vi "RunMeOld.vi"() -> ()   [LabVIEW 2011]
doc: "Use this template to create an application that executes repeatedly until you click the Stop button. This template polls the state of the Stop button and does not use events. Use the Top-Level Application template (not available in the Base package) to create a single-loop application with event handling."
uses:
  Instance           1 33Saved   SingleLoopApplication.vit .vi
  <vilib>/Instr/_visa.llb/VISA Configure Serial Port (Instr).vi
  <vilib>/gmath/NI_Gmath.lvlib
  <vilib>/gmath/NumericalOptimization/Nonlinear Curve Fit LM formula string.vi
panel:
  out "Position":dbl(knob) max=500.0 scale=0.0..360.0
  out "Measurement OK":bool
  out "Residuals":cluster{u32[], dbl[]}(graph)
  out "Instant data":cluster{"velocity":dbl, "position":u32}
  in  "initial parameters":dbl[](array[numeric])=[1.0, 1.0, 1.0]
  out "best fit parameters":dbl[](array[numeric])
  in  "model description":T1={"model"="r+n*sin(x/500*2*3.141593+f)", "Parameters"=["r", "n", "f"], "x"="x"}
  in  "Clear":bool
  in  "index (page)":i32
  out "Previus measurements":cluster{u32[], "best nonlinear fit":dbl[]}[](graph)
  out "Current measurement":cluster{u32[], dbl[]}(graph)
  out "home?":bool=TRUE
  in  "Motor on":bool
  in  "Connect":bool
  in  "VISA resource name":refnum<visa-resource-name>="COM5"
  out "error out":errorcluster
  in  "stop":bool
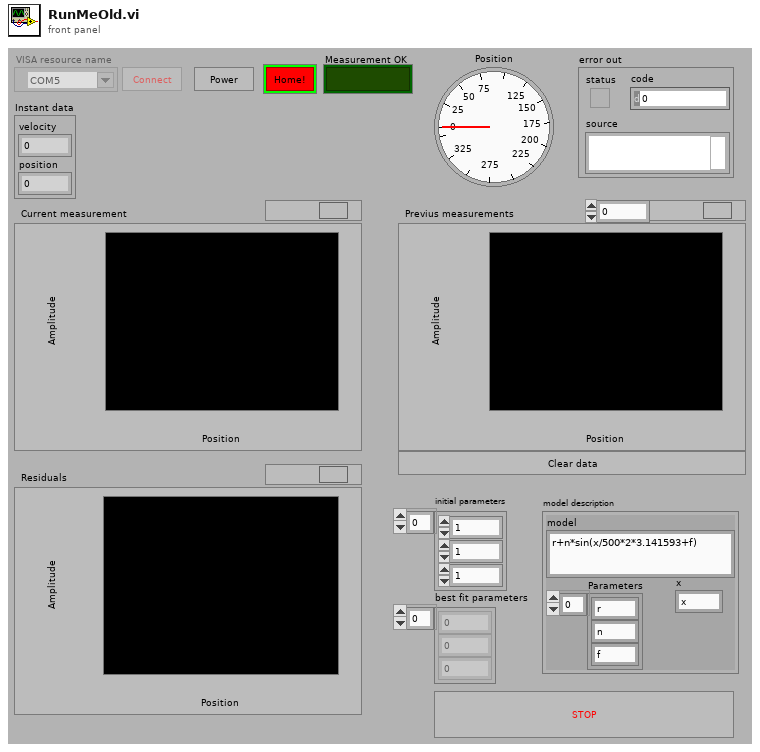
[diagram p1: front panel]
types:
  T1 = cluster{"model":string, "Parameters":string[], "x":string}
  T2 = enum8{"Enabled", "Disabled", "Disabled and Grayed Out"}
  T3 = cluster{"velocity":dbl, "position":u32, "home?":bool, "reset?":bool, "angle":dbl, "new?":bool}
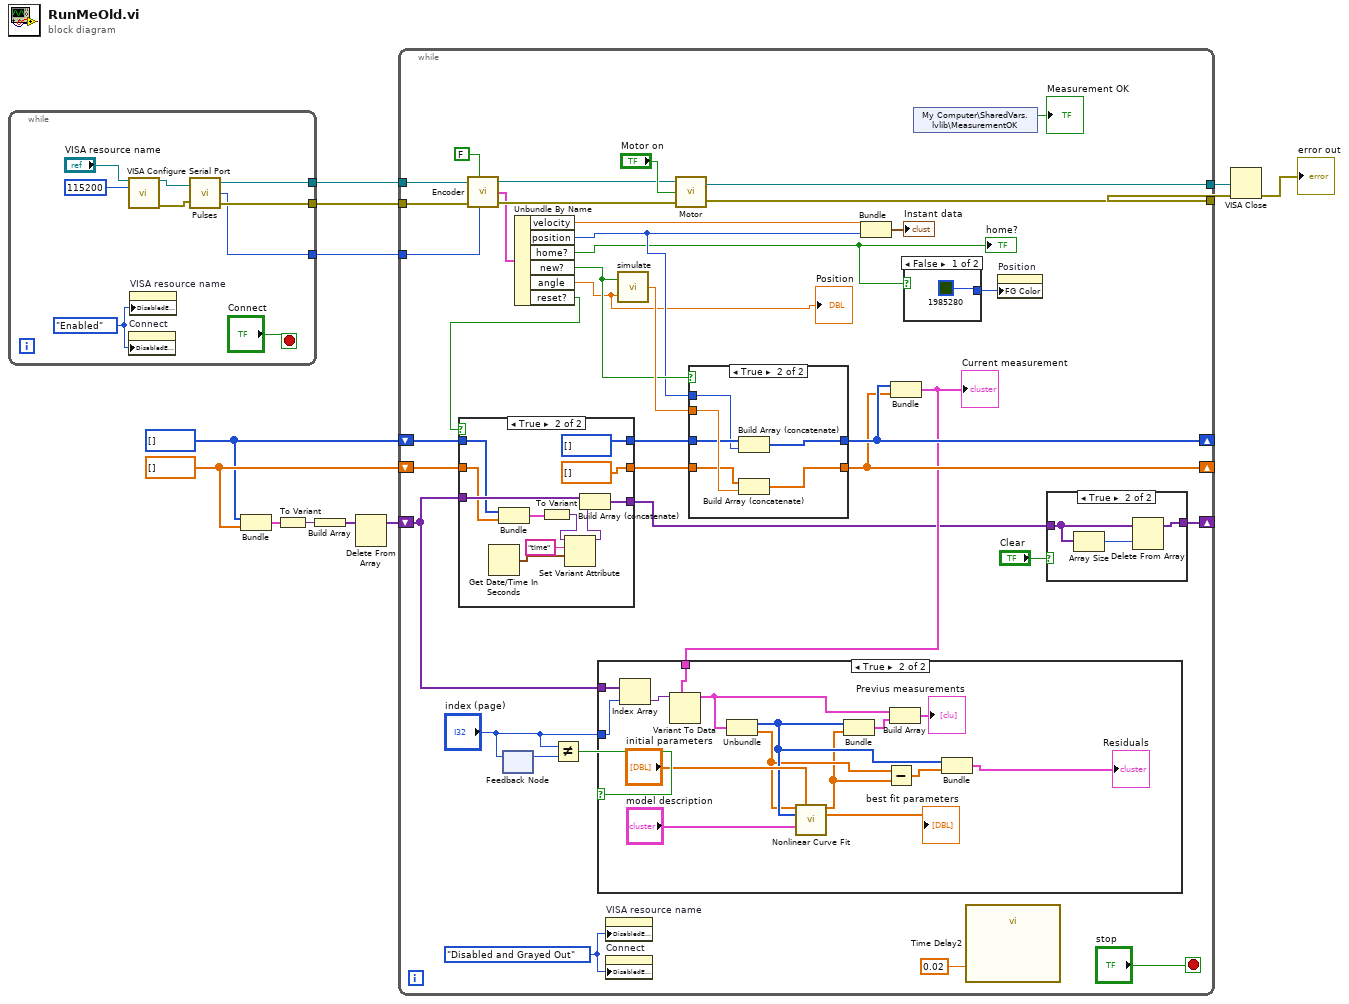
[diagram p0: block diagram]
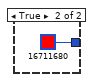
[diagram p2: hidden frame]
diagram:
  w6 = u32[] []
  w7 = dbl[] []
  n1 = while {
    tunnel: [w16] -> w2
    tunnel: [w15] -> w11
    tunnel: [w13] -> w1
    stop <- "Connect" stop-if-true
    w18 = T2."Enabled" ("Disabled")
    n2 = call-poly "VISA Configure Serial Port"("VISA resource name"="VISA resource name", "baud rate (9600)"=u32 115200) -> ("VISA resource name out"=w17:refnum<visa-resource-name>, "error out"=w14:errorcluster)  [unwired: 12 in]
    n3 = property on="Connect" class="Bool"("DisabledEnum"=w18) -> ()  [unwired: 2 in, 2 out]
    n4 = property on="VISA resource name" class="VISAName"("DisabledEnum"=w18) -> ()  [unwired: 2 in, 2 out]
    n5 = call "Pulses.vi"("error in (no error)"=w14, "VISA resource name in"=w17) -> ("error out"=w15:errorcluster, "pulses"=w13:u32, "VISA resource name out"=w16:refnum<visa-resource-name>)
  }
  n6 = Bundle(w6, w7) -> (w8:cluster{u32[], dbl[]})  [unwired: 1 in]
  n7 = To Variant(anything=w8) -> (Variant=w5:variant)
  n8 = Build Array(w5) -> (w4:variant[])
  n9 = Delete From Array(array=w4) -> (array with subset deleted=w3:variant[])  [unwired: 2 in, 1 out]
  n10 = while {
    tunnel: [w48] -> w12
    tunnel: w2 -> [w57]
    tunnel: w11 -> [w56]
    tunnel: [w50] -> w10
    shift-right: [w38] -> _
    shift-left: w7 -> [w41]
    shift-right: [w35] -> _
    shift-left: w3 -> [w47]
    shift-right: [w39] -> _
    shift-left: w6 -> [w42]
    tunnel: w1 -> [w27]
    stop <- "stop" stop-if-true
    w55 = T2."Disabled and Grayed Out" ("Disabled")
    n11 = call "Encoder.vi"("Serial Port in"=w57, "simulate?"=FALSE, "error in"=w56, "pulses"=w27) -> ("Serial Port out"=w49:refnum<visa-resource-name>, "status"=w45:T3, "error out"=w51:errorcluster)  [unwired: 1 in]
    n12 = feedback-in #1("index (page)") -> ()
    n13 = feedback #1() -> (w33:i32)  [unwired: 1 in]
    n14 = Unbundle By Name(w45) -> ("velocity"=w46:dbl, "position"=w25:u32, "home?"=w22:bool, "new?"=w29:bool, "angle"=w24:dbl, "reset?"=w30:bool)
    "home?" <- w22
    "Position" <- w24
    n15 = case shown="True" w30 {
      tunnel: w42 -> [w90 w99]
      tunnel: [w90 u32[] []] -> w44
      tunnel: [w89 w100] -> w36
      tunnel: w47 -> [w89 w101]
      tunnel: w41 -> [w88 w98]
      tunnel: [w88 dbl[] []] -> w40
      frame False {
      }
      frame True {
        n16 = Get Date/Time In Seconds() -> (seconds since 1Jan1904=w93:timestamp)
        n17 = Bundle(w99, w98) -> (w97:cluster{u32[], dbl[]})  [unwired: 1 in]
        n18 = To Variant(anything=w97) -> (Variant=w94:variant)
        n19 = Set Variant Attribute(Variant=w94, name="time", value=w93) -> (Variant out=w91:variant)  [unwired: 1 in, 2 out]
        n20 = Build Array (concatenate)(w101, w91) -> (w100:variant[])
      }
    }
    n21 = Not Equal?(x="index (page)", y=w33) -> (x != y?=w31:bool)
    n22 = property on="VISA resource name" class="VISAName"("DisabledEnum"=w55) -> ()  [unwired: 2 in, 2 out]
    n23 = property on="Connect" class="Bool"("DisabledEnum"=w55) -> ()  [unwired: 2 in, 2 out]
    n24 = call "simulate.vi"("angle"=w24, "initialize"=w29) -> ("mean"=w43:dbl)  [unwired: 2 out]
    n25 = call "Motor.vi"("error in"=w51, "Motor on?"="Motor on", "Serial Port in"=w49) -> ("error out"=w50:errorcluster, "Serial Port out"=w48:refnum<visa-resource-name>)
    n26 = case shown="True" w29 {
      tunnel: w44 -> [w81 w85]
      tunnel: w43 -> [_ w87]
      tunnel: [w81 w83] -> w39
      tunnel: w25 -> [_ w84]
      tunnel: w40 -> [w80 w86]
      tunnel: [w80 w82] -> w38
      frame False {
      }
      frame True {
        n27 = Build Array (concatenate)(w85, w84) -> (w83:u32[])
        n28 = Build Array (concatenate)(w86, w87) -> (w82:dbl[])
      }
    }
    n29 = Bundle("velocity"=w46, "position"=w25) -> (→"Instant data":cluster{"velocity":dbl, "position":u32})  [unwired: 1 in]
    n30 = Bundle(w39, w38) -> (w37:cluster{u32[], dbl[]})  [unwired: 1 in]
    "Current measurement" <- w37
    n31 = case shown="True" w31 {
      tunnel: w47 -> [_ w75]
      tunnel: w37 -> [_ w73]
      tunnel: "index (page)" -> [_ w69]
      frame False {
      }
      frame True {
        n32 = Index Array(array=w75, index=w69) -> (element=w74:variant)
        n33 = Variant To Data(type=w73, Variant=w74) -> (data=w68:cluster{u32[], dbl[]})  [unwired: 1 in, 1 out]
        n34 = Unbundle(w68) -> (w65:u32[], w63:dbl[])
        n35 = call-poly <vilib>:"Nonlinear Curve Fit.vi"("Y"=w63, "initial parameters"="initial parameters", "X"=w65, "model description"="model description") -> ("best nonlinear fit"=w62:dbl[], "best fit parameters"=→"best fit parameters":dbl[])  [unwired: 7 in, 3 out]
        n36 = Bundle(w65, "best nonlinear fit"=w62) -> (w67:cluster{u32[], "best nonlinear fit":dbl[]})  [unwired: 1 in]
        n37 = Subtract(x=w63, y=w62) -> (x-y=w64:dbl[])
        n38 = Build Array(w68, w67) -> (→"Previus measurements":cluster{u32[], "best nonlinear fit":dbl[]}[])
        n39 = Bundle(w65, w64) -> (→"Residuals":cluster{u32[], dbl[]})  [unwired: 1 in]
      }
    }
    n40 = case shown="False" w22 {
      tunnel: [u32 1985280 u32 16711680] -> w23
      frame False {
      }
      frame True {
      }
    }
    n41 = shared-variable "My Computer\\SharedVars.lvlib\\MeasurementOK"() -> (→"Measurement OK":bool)  [unwired: 1 in, 1 out]
    n42 = call "Time Delay2"("Delay Time (s)"=0.02) -> ()  [unwired: 10 in, 1 out]
    n43 = property on="Position" class="Knob (strict)"("FG Color"=w23) -> ()  [unwired: 2 in, 2 out]
    n44 = case shown="True" "Clear" {
      tunnel: w36 -> [w76 w78]
      tunnel: [w76 w77] -> w35
      frame False {
      }
      frame True {
        n45 = Array Size(array=w78) -> (size(s)=w79:i32)
        n46 = Delete From Array(array=w78, length=w79) -> (array with subset deleted=w77:variant[])  [unwired: 1 in, 1 out]
      }
    }
  }
  n47 = VISA Close(VISA resource name=w12, error in (no error)=w10) -> (error out=→"error out":errorcluster)
